vi "NN Example.vi"() -> ()   [LabVIEW 2024]
panel:
  out "Numeric":i32
  out "Waveform Chart":dbl(graph)
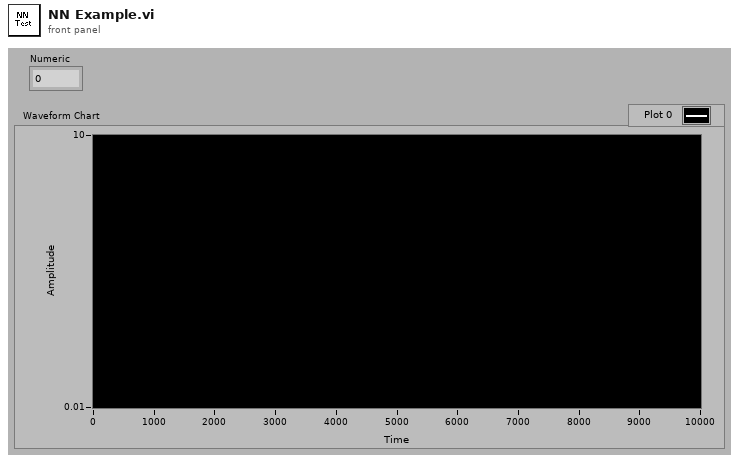
[diagram p1: front panel]
types:
  T1 = typedef "NeuronData.ctl" = cluster{"Neuron Layer":cluster{"Weights":dbl[], "Y Calc":dbl, "Delta Error":dbl}[]}[]
  T2 = cluster{"Neuron Layer":cluster{"Weights":dbl[], "Y Calc":dbl, "Delta Error":dbl}[]}
  T3 = cluster{"Weights":dbl[], "Y Calc":dbl, "Delta Error":dbl}[]
  T4 = cluster{"Weights":dbl[], "Y Calc":dbl, "Delta Error":dbl}
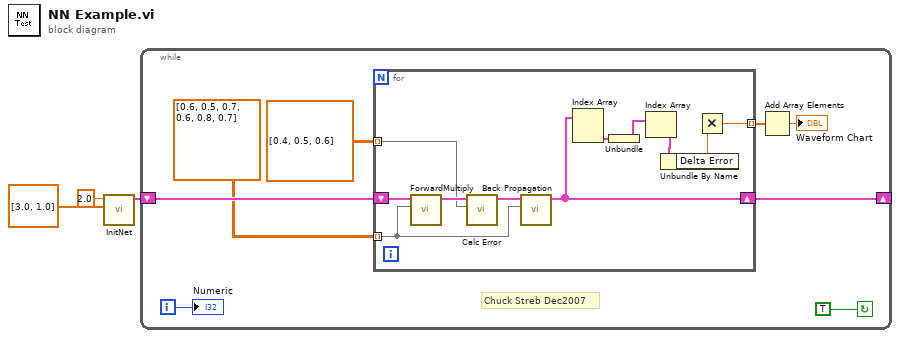
[diagram p0: block diagram]
diagram:
  n1 = call "InitNet.vi"("Hidden Neurons"=dbl[] [3.0, 1.0], "Inputs"=2.0) -> ("Neuron Stucture"=w1:T1)  [unwired: 9 in]
  n2 = while {
    shift-right: [w9] -> _
    shift-left: w1 -> [w11]
    i -> [w4]
    stop <- TRUE continue-if-true
    # "Chuck Streb Dec2007"
    n3 = for {
      tunnel: dbl[][] [[0.6, 0.5], [0.7, 0.6], [0.8, 0.7]] ("Inputs") -> [w14] mode=indexing
      tunnel: dbl[][] [[0.4], [0.5], [0.6]] ("Inputs") -> [w15] mode=indexing
      shift-right: [w19] -> w9
      shift-left: w11 -> [w22]
      tunnel: [w12] -> w6 mode=indexing
      n4 = call "ForwardMultiply.vi"("Inputs"=w14, "Neuron Stucture In"=w22) -> ("Neuron Stucture Out"=w21:T1)  [unwired: 8 in, 1 out]
      n5 = call "Calc Error.vi"("YInput"=w15, "Neuron Stucture In"=w21) -> ("Neuron Stucture Out"=w20:T1)  [unwired: 9 in]
      n6 = call "Back Propagation.vi"("X Input"=w14, "Neuron Stucture In"=w20) -> ("Neuron Stucture Out"=w19:T1)  [unwired: 9 in]
      n7 = Index Array(array=w19) -> (element #2=w18:T2)  [unwired: 2 in, 1 out]
      n8 = Unbundle(w18) -> ("Neuron Layer"=w17:T3)
      n9 = Index Array(array=w17) -> (element=w16:T4)  [unwired: 1 in]
      n10 = Unbundle By Name(w16) -> ("Delta Error"=w13:dbl)
      n11 = Multiply(x=w13, y=w13) -> (x*y=w12:dbl)
    }
    n12 = Add Array Elements(numeric array=w6) -> (sum=→"Waveform Chart":dbl)
    "Numeric" <- w4
  }
